vi "Unescape_Json.vi"(10 "Json_String":string) -> (3 "String":string)   [LabVIEW 2019]
panel:
  # "Unscape offending characters \\ \\n \\t\""
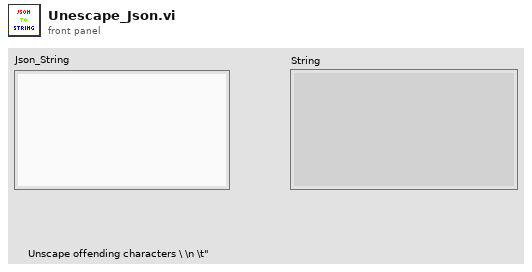
[diagram p1: front panel]
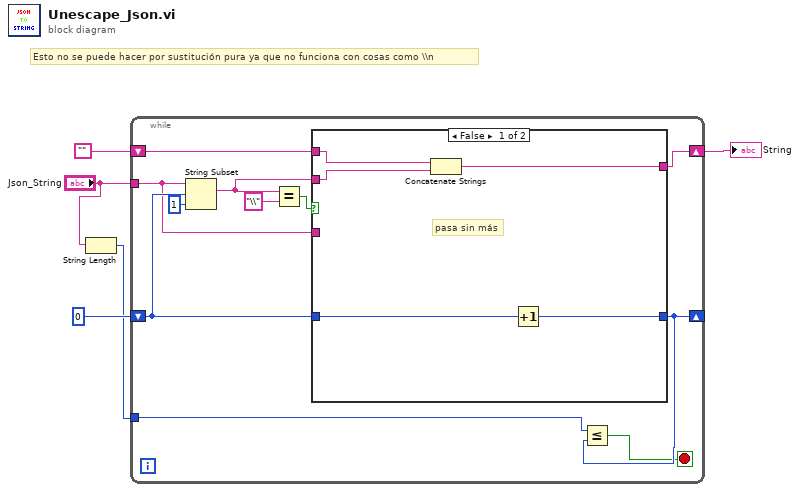
[diagram p0: block diagram]
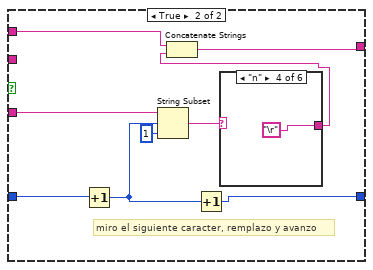
[diagram p2: hidden frame]
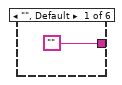
[diagram p3: hidden frame]
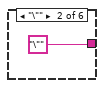
[diagram p4: hidden frame]
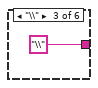
[diagram p5: hidden frame]
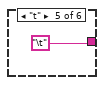
[diagram p6: hidden frame]
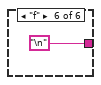
[diagram p7: hidden frame]
diagram:
  # "Esto no se puede hacer por sustitución pura ya que no funciona con cosas como \\\\n"
  n1 = String Length(string="Json_String") -> (length=w1:i32)
  n2 = while {
    shift-right: [w10] -> w4
    shift-left: "" -> [w11]
    tunnel: "Json_String" -> [w9]
    shift-right: [w7] -> _
    shift-left: 0 -> [w12]
    tunnel: w1 -> [w8]
    stop <- w6 stop-if-true
    n3 = String Subset(string=w9, offset (0)=w12, length (rest)=1 ("length (rest)")) -> (substring=w14:string)
    n4 = Equal?(x=w14, y="\\") -> (x = y?=w15:bool)
    n5 = case shown="False" w15 {
      tunnel: w14 -> [w18 _]
      tunnel: w12 -> [w21 w29]
      tunnel: [w20 w23] -> w7
      tunnel: w11 -> [w19 w26]
      tunnel: [w17 w25] -> w10
      tunnel: w9 -> [_ w28]
      frame False {
        # "pasa sin más"
        n6 = Concatenate Strings(w19, w18) -> (w17:string)
        n7 = Increment(x=w21) -> (x+1=w20:i32)
      }
      frame True {
        # "miro el siguiente caracter, remplazo y avanzo"
        n8 = Increment(x=w29) -> (x+1=w24:i32)
        n9 = String Subset(string=w28, offset (0)=w24, length (rest)=1 ("length (rest)")) -> (substring=w27:string)
        n10 = Increment(x=w24) -> (x+1=w23:i32)
        n11 = case shown="\"n\"" w27 {
          tunnel: ["" "\"" "\\" ("y") "\r" "\t" "\n"] -> w22
          frame "", Default {
          }
          frame "\"" {
          }
          frame "\\" {
          }
          frame "n" {
          }
          frame "t" {
          }
          frame "f" {
          }
        }
        n12 = Concatenate Strings(w26, w22) -> (w25:string)
      }
    }
    n13 = Less Or Equal?(x=w8, y=w7) -> (x <= y?=w6:bool)
  }
  "String" <- w4
